vi "Can Move To.vi"(10 "Room in":string[](array[string]), 11 "Amphipod Type in":string) -> (1 "Can Move To?":bool, 2 "Room out":string[](array[string]), 3 "Amphipod Type out":string)   [LabVIEW 2019, in "23.lvlib" / "State.lvclass"]
uses:
  State.lvclass
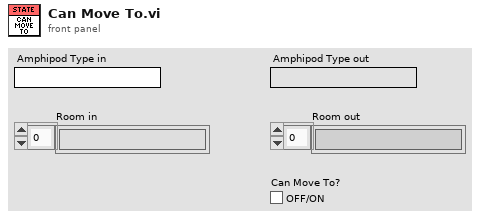
[diagram p1: front panel]
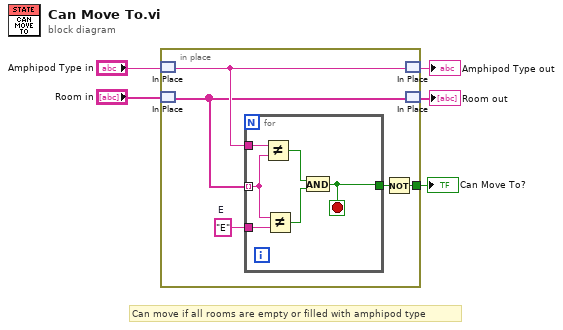
[diagram p0: block diagram]
diagram:
  # "Can move if all rooms are empty or filled with amphipod type"
  n1 = in-place {
    in-place-border: [w8] -> w5
    w10 = "E"  # E
    n2 = in-place-match #1("Amphipod Type in") -> (w7:string)
    n3 = in-place-match #2("Room in") -> (w6:string[])
    n4 = for {
      tunnel: w6 -> [w15] mode=indexing
      tunnel: w7 -> [w16]
      tunnel: w10 -> [w14]
      tunnel: [w11] -> w9
      stop <- w11 stop-if-true
      n5 = Not Equal?(x=w16, y=w15) -> (x != y?=w13:bool)
      n6 = Not Equal?(x=w15, y=w14) -> (x != y?=w12:bool)
      n7 = And(x=w13, y=w12) -> (x .and. y?=w11:bool)
    }
    n8 = Not(x=w9) -> (.not. x?=w8:bool)
    n9 = in-place-match #1(w7) -> (→"Amphipod Type out":string)
    n10 = in-place-match #2(w6) -> (→"Room out":string[])
  }
  "Can Move To?" <- w5
